vi "New dotNET SSL Server Socket.vi"(8 "error in (no error)":errorcluster, 11 ".NET TcpClient":refnum<k24>) -> (0 "error out":errorcluster, 3 "dotNET SSL Socket out":refnum<class "dotNET SSL Server.lvclass">)   [LabVIEW 2013, in "dotNET SSL Socket.lvlib" / "dotNET SSL Server.lvclass"]
uses:
  dotNET SSL Server/dotNET SSL Server.lvclass
  dotNET SSL Socket.lvclass/dotNET SSL Socket.ctl
  Write SSLStream.vi
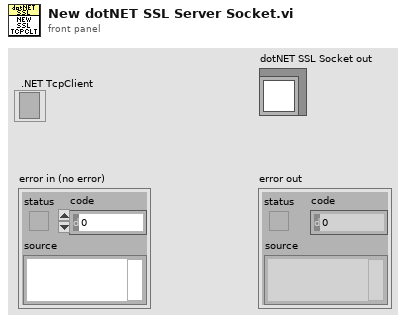
[diagram p1: front panel]
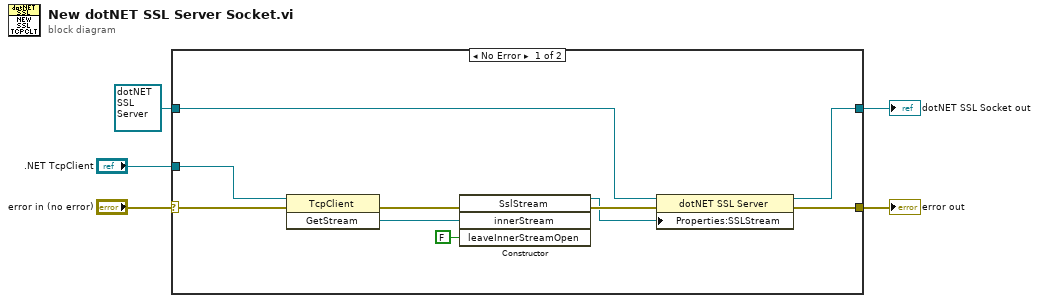
[diagram p0: block diagram]
diagram:
  n1 = case shown="No Error" "error in (no error)" {
    selector: "error in (no error)" -> [w11 w17]
    tunnel: [w9 w17] -> w4
    tunnel: [w6 w16] -> w2
    tunnel: refnum<class "dotNET SSL Server.lvclass"> refnum ("dotNET SSL Socket in") -> [w7 w16]
    tunnel: ".NET TcpClient" -> [w8 _]
    frame No Error {
      n2 = invoke class="TcpClient" method="GetStream"(reference=w8, error in=w11) -> (error out=w13:errorcluster, "GetStream"=w15:refnum<k24>)  [unwired: 1 in, 1 out]
      n3 = constructor class="SslStream"(error in=w13, "innerStream"=w15, "leaveInnerStreamOpen"=FALSE) -> (reference out=w10:refnum<k24>, error out=w12:errorcluster)  [unwired: 2 in, 3 out]
      n4 = property class="dotNET SSL Server"(reference=w7, error in=w12, "Properties:SSLStream"=w10) -> (reference out=w6:refnum<class "dotNET SSL Server.lvclass">, error out=w9:errorcluster)
    }
    frame Error {
    }
  }
  "error out" <- w4
  "dotNET SSL Socket out" <- w2
